vi "port.vi"() -> ()   [LabVIEW 2013]
panel:
  in  "port":u16
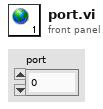
[diagram p1: front panel]
diagram:
